vi "Control Type.vi"(11 "Valve in":refnum<class "ValueSetControl.lvclass">) -> (2 "Valve Type":string)   [LabVIEW 2020, in "VolatusControl.lvlib" / "ValueSetControl.lvclass"]
uses:
  ValueSetControl.lvclass
  ValueSetControl.lvclass/ValueSetControl.ctl
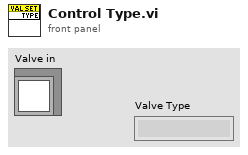
[diagram p1: front panel]
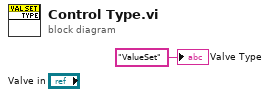
[diagram p0: block diagram]
diagram:
  "Valve Type" <- "ValueSet" ("Valve Type")
